vi "Gen IOP Filter.vi"(10 "Cutoff Freq":dbl) -> (1 "num_HP":dbl[](array[numeric]), 2 "num_LP":dbl[](array[numeric]))   [LabVIEW 2016]
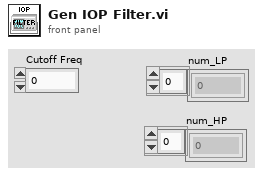
[diagram p1: front panel]
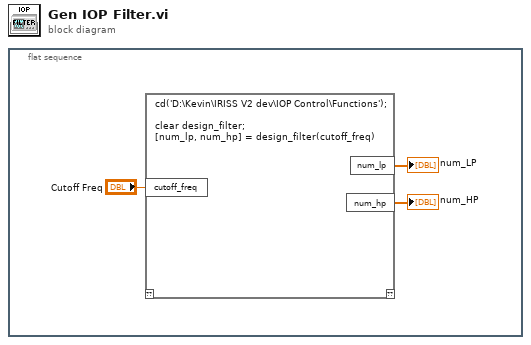
[diagram p0: block diagram]
diagram:
  n1 = flat-sequence {
    frame #0 {
      n2 = script code="cd('D:\\Kevin\\IRISS V2 dev\\IOP Control\\Functions');\n\nclear design_filter;\n[num_lp, num_hp] = design_filter(cutoff_freq)"("cutoff_freq"="Cutoff Freq") -> ("num_hp"=→"num_HP":dbl[], "num_lp"=→"num_LP":dbl[])  [unwired: 1 in, 1 out]
    }
  }
